vi "Refresh Timer.vi"(8 "error in (no error)":errorcluster, 11 "Motions in":refnum<class "Motions.lvclass">) -> (0 "error out":errorcluster, 3 "Motions out":refnum<class "Motions.lvclass">)   [LabVIEW 2016, in "Hardware.lvlib" / "Motions.lvlib" / "Motions.lvclass"]
uses:
  <userlib>/Common Components/Hardware/Abstract System/Motions/Motions/Motions.lvclass
  <userlib>/Common Components/Hardware/Abstract System/Motions/Motions/Motions.lvclass/Motions.ctl
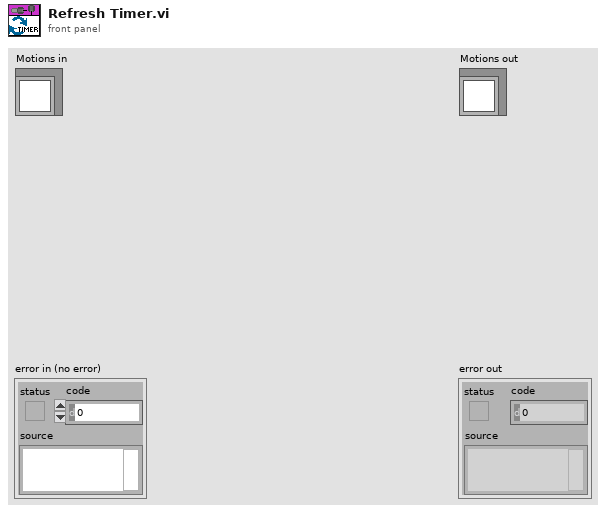
[diagram p1: front panel]
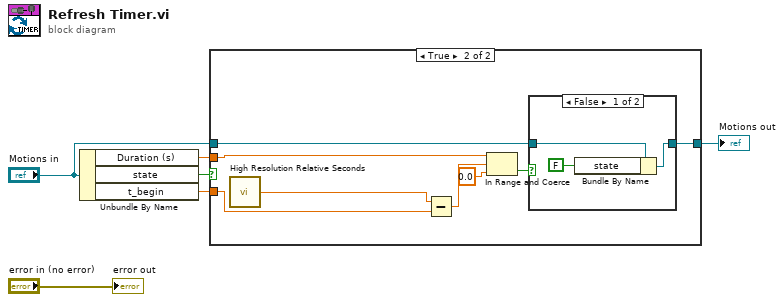
[diagram p0: block diagram]
diagram:
  n1 = Unbundle By Name("Motions in") -> ("Duration (s)"=w1:dbl, "state"=w5:bool, "t_begin"=w4:dbl)
  n2 = case shown="True" w5 {
    tunnel: w4 -> [_ w14]
    tunnel: w1 -> [_ w9]
    tunnel: "Motions in" -> [w7 w12]
    tunnel: [w7 w11] -> w2
    frame False {
    }
    frame True {
      n3 = call <vilib>:"High Resolution Relative Seconds.vi"() -> ("relative seconds"=w15:dbl)
      n4 = Subtract(x=w15, y=w14) -> (x-y=w10:dbl)
      n5 = In Range and Coerce(upper limit=w9, x=w10, lower limit=0.0) -> (In Range?=w13:bool)  [unwired: 1 out]
      n6 = case shown="False" w13 {
        tunnel: w12 -> [w18 w19]
        tunnel: [w17 w19] -> w11
        frame False {
          n7 = Bundle By Name(cluster=w18, "state"=FALSE ("Timer.state")) -> (w17:refnum<class "Motions.lvclass">)
        }
        frame True {
        }
      }
    }
  }
  "Motions out" <- w2
  "error out" <- "error in (no error)"
